vi "sv_Subset Filter Design.vi"(0 "fs":dbl=1.0 format="%.2f", 1 "filter type":T1(ring), 5 "fl":dbl=0.05 format="%.2f", 7 "fh":dbl=0.25 format="%.2f", 9 "delta f":dbl=0.1 format="%.2f", 11 "A stop [dB]":dbl=72.0 format="%.2f") -> (4 "filter coefficients":dbl[](array[numeric]) format="%.2f", 6 "taps":i32, 15 "error":i32)   [LabVIEW 2017, in "SoundVib_ContSweptSine.lvlib"]
uses:
  <vilib>/addons/Sound and Vibration/svt_Continuous Swept Sine/SoundVib_ContSweptSine.lvlib
  <vilib>/addons/Sound and Vibration/Order Analysis/Resample Order Tracking/SoundVib_Resampling.lvlib
  <vilib>/Analysis/NI_AALBase.lvlib
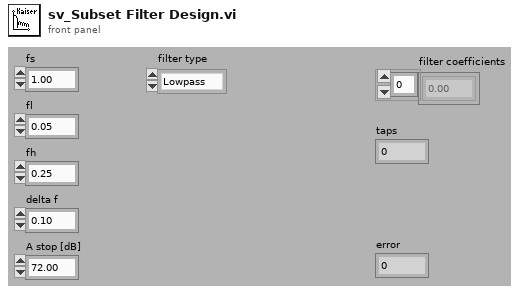
[diagram p1: front panel]
types:
  T1 = enum32{"Lowpass", "Highpass", "Bandpass", "Bandstop"}
  T2 = enum32{"None", "Hanning", "Hamming", "Triangular", "Blackman", "Exact Blackman", "Blackman-Harris", "Kaiser-Bessel", "Flat Top"}
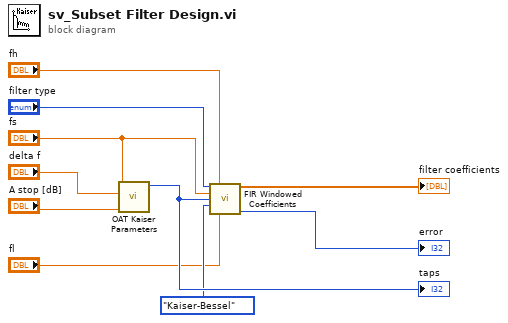
[diagram p0: block diagram]
diagram:
  n1 = call <vilib>:"OAT Kaiser Parameters.vi"("A stop [dB]"="A stop [dB]", "delta f"="delta f", "fs"="fs") -> ("taps"=w8:i32)  [unwired: 7 in, 1 out]
  "taps" <- w8
  n2 = call <vilib>:"FIR Windowed Coefficients.vi"("filter type"="filter type", "high cutoff freq: fh"="fh", "sampling freq: fs"="fs", "taps"=w8, "window"=T2."Kaiser-Bessel", "low cutoff freq: fl"="fl") -> ("FIR Windowed Coefficients"=→"filter coefficients":dbl[], "error"=→"error":i32)  [unwired: 8 in]
